vi "Write Speed.vi"(8 "error in (no error)":errorcluster, 10 "Speed":dbl[unit]=5e-09, 11 "Stepper.lvclass in":refnum<class "Stepper.lvclass">) -> (0 "error out":errorcluster, 3 "Stepper.lvclass out":refnum<class "Stepper.lvclass">)   [LabVIEW 2009, in "Stepper.lvclass"]
uses:
  Stepper.lvclass
  Stepper.lvclass/Stepper.ctl
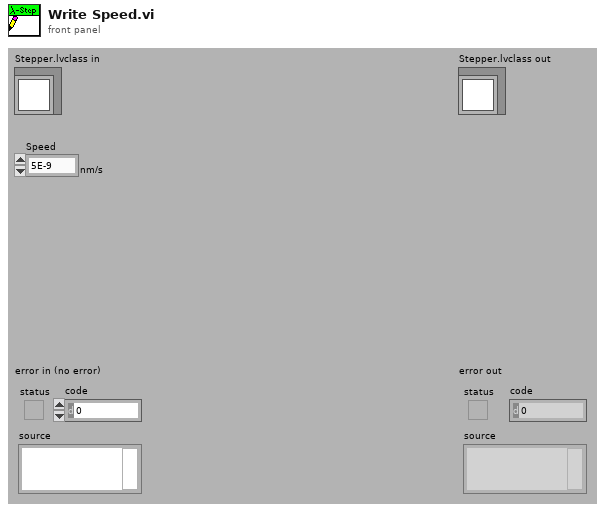
[diagram p1: front panel]
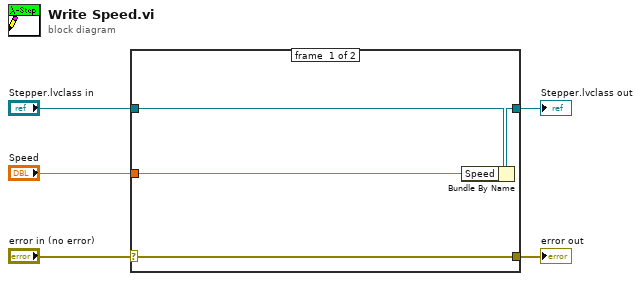
[diagram p0: block diagram]
diagram:
  n1 = case shown="No Error" "error in (no error)" {
    selector: "error in (no error)" -> [w9 w10]
    tunnel: [w9 w10] -> w4
    tunnel: [w7 w11] -> w2
    tunnel: "Stepper.lvclass in" -> [w8 w11]
    tunnel: "Speed" -> [w6 _]
    frame #0 {
      n2 = Bundle By Name(cluster=w8, "Speed"=w6) -> (w7:refnum<class "Stepper.lvclass">)
    }
    frame #1 {
    }
  }
  "error out" <- w4
  "Stepper.lvclass out" <- w2
